vi "Configure Processes.vi"(8 "error in (no error)":errorcluster, 10 "Processes":string[](array[string]), 11 "Debugger In":refnum<class "Debugger.lvclass">) -> (0 "error out":errorcluster, 3 "Debugger Out":refnum<class "Debugger.lvclass">)   [LabVIEW 2020, in "Debugger.lvclass"]
uses:
  Debugger.lvclass
  C:/Users/anton/Documents/GitHub/triarc-debugger/source/Process/Debug Process.lvclass
  Process/Debug Process.lvclass/Debug Process.ctl
  <vilib>/Utility/error.llb/Clear Errors.vi
  Filter by Process/Filter by Process.lvclass
  C:/Users/anton/Documents/GitHub/triarc-debugger/source/Filter/Filter.lvclass
  <vilib>/Utility/error.llb/Error Cluster From Error Code.vi
  Debugger.lvclass/Debugger.ctl
  Process/Debug Process.lvclass
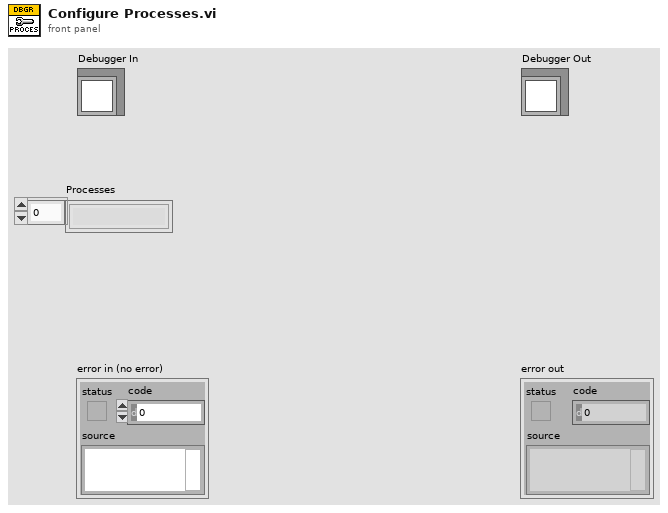
[diagram p1: front panel]
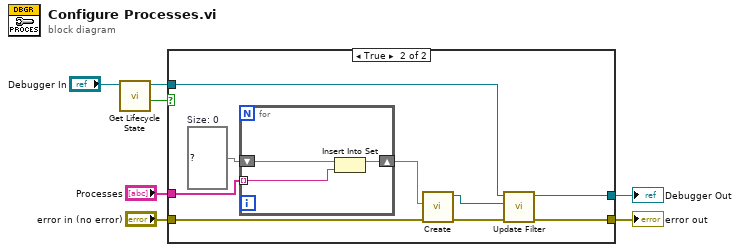
[diagram p0: block diagram]
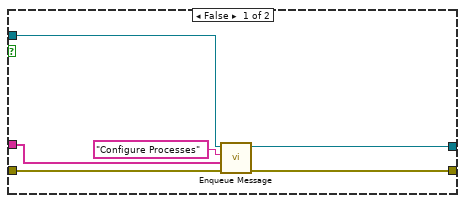
[diagram p2: hidden frame]
diagram:
  n1 = call "Get Lifecycle State.vi"("Process In"="Debugger In") -> ("In Process Loop?"=w1:bool, "Process Out"=w2:refnum<class "Debugger.lvclass">)  [unwired: 7 in, 2 out]
  n2 = case shown="True" w1 {
    tunnel: "error in (no error)" -> [w13 w19]
    tunnel: [w12 w18] -> w6
    tunnel: [w11 w21] -> w4
    tunnel: "Processes" -> [w9 w20]
    tunnel: w2 -> [w8 w22]
    frame False {
      n3 = call "Enqueue Message.vi"("error in (no error)"=w13, "Message Data"=w9, "Message"="Configure Processes", "Process In"=w8) -> ("error out"=w12:errorcluster, "Process Out"=w11:refnum<class "Debugger.lvclass">)  [unwired: 6 in]
    }
    frame True {
      w16 = set{string} {}  # Size: 0
      n4 = for {
        shift-right: [w24] -> w17
        shift-left: w16 -> [w25]
        tunnel: w20 -> [w23] mode=indexing
        n5 = Insert Into Set(10:w23, 11:w25) -> (3:w24:set{string})  [unwired: 1 out]
      }
      n6 = call "Create.vi"("error in (no error)"=w19, "Processes"=w17) -> ("error out"=w14:errorcluster, "Filter by Process out"=w15:refnum<class "Filter by Process.lvclass">)  [unwired: 8 in]
      n7 = call "Update Filter.vi"("error in (no error)"=w14, "Filter in"=w15, "Debugger in"=w22) -> ("error out"=w18:errorcluster, "Debugger out"=w21:refnum<class "Debugger.lvclass">)  [unwired: 7 in]
    }
  }
  "error out" <- w6
  "Debugger Out" <- w4
